vi "TimeInterpPose2d_CleanUp.vi"(11 "in TimeInterpPose":T1 {"Pose"."ROTATION"."SIN" format="%13.4f"; "Pose"."ROTATION"."COS" format="%13.4f"; "Pose"."ROTATION"."VALUE" format="%13.4f"; "Pose"."TRANSLATION"."Y" format="%14.3f"; "Pose"."TRANSLATION"."X" format="%14.3f"}) -> (0 "Error":bool, 3 "out TimeInterpPose":T1 {"Pose"."ROTATION"."SIN" format="%13.4f"; "Pose"."ROTATION"."COS" format="%13.4f"; "Pose"."ROTATION"."VALUE" format="%13.4f"; "Pose"."TRANSLATION"."Y" format="%14.3f"; "Pose"."TRANSLATION"."X" format="%14.3f"})   [LabVIEW 2019, in "Trajectory_Library.lvlib"]
doc: "Removes samples older than our current history size.\n\nInputs:\n - In TimeInterpPose2d -- Input data cluster.\n\nOutputs:\n - Out TimeInterpPose2d -- Updated data cluster.\n - Error -- Returns TRUE if an error occured."
uses:
  Trajectory_Library.lvlib
  TIME_INTERPOLATABLE_POSE2D.ctl
  POSE2D.ctl
  TRANSLATION2D.ctl
  ROTATION2D.ctl
  <vilib>/gmath/NI_Gmath.lvlib
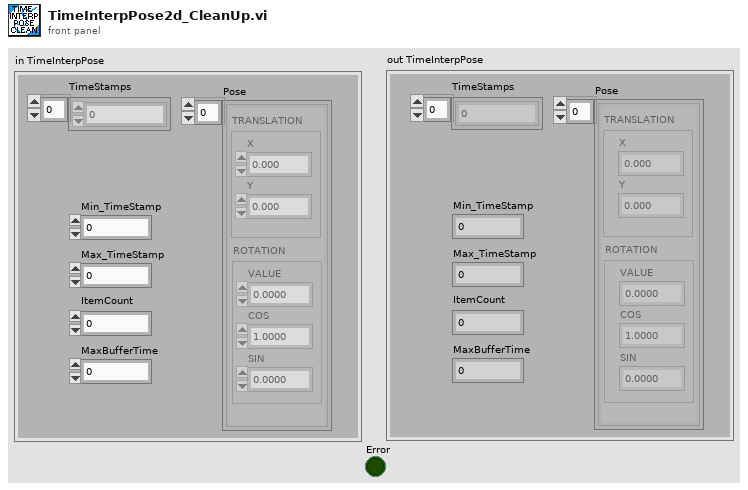
[diagram p1: front panel]
types:
  T1 = typedef "Trajectory_Library.lvlib/TIME_INTERPOLATABLE_POSE2D.ctl" = cluster{"TimeStamps":dbl[], "Pose":T2[], "Min_TimeStamp":dbl, "Max_TimeStamp":dbl, "ItemCount":i32, "MaxBufferTime":dbl}
  T2 = typedef "Trajectory_Library.lvlib/POSE2D.ctl" = cluster{"TRANSLATION":T3, "ROTATION":T4}
  T3 = typedef "Trajectory_Library.lvlib/TRANSLATION2D.ctl" = cluster{"X":dbl, "Y":dbl}
  T4 = typedef "Trajectory_Library.lvlib/ROTATION2D.ctl" = cluster{"VALUE":dbl, "COS":dbl, "SIN":dbl}
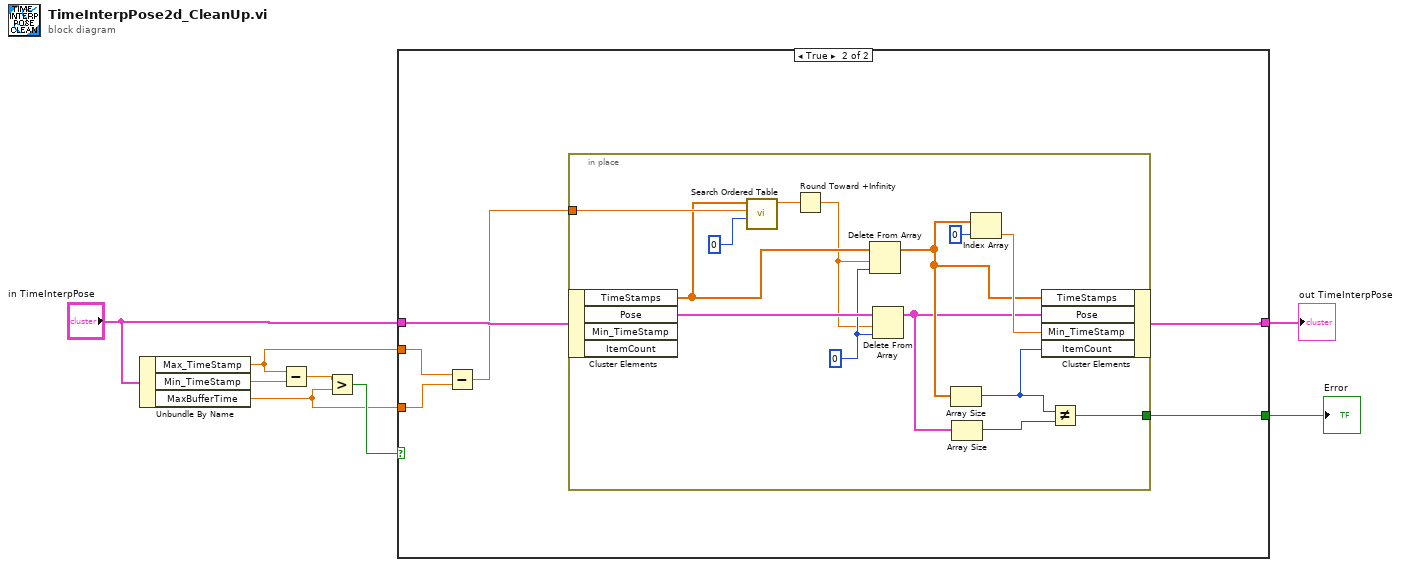
[diagram p0: block diagram]
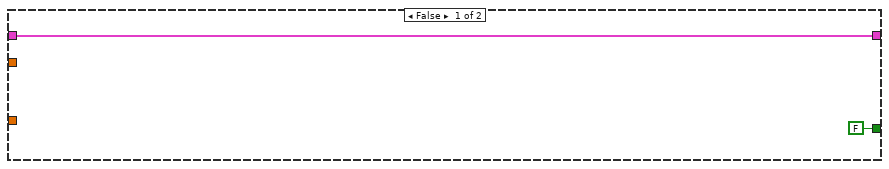
[diagram p2: hidden frame]
diagram:
  n1 = Unbundle By Name("in TimeInterpPose") -> ("Max_TimeStamp"=w3:dbl, "Min_TimeStamp"=w6:dbl, "MaxBufferTime"=w2:dbl)
  n2 = Subtract(x=w3, y=w6) -> (x-y=w5:dbl)
  n3 = Greater?(x=w5, y=w2) -> (0:w4:bool)
  n4 = case shown="True" w4 {
    tunnel: "in TimeInterpPose" -> [w10 w14]
    tunnel: [w10 w12] -> w8
    tunnel: w3 -> [_ w16]
    tunnel: w2 -> [_ w15]
    tunnel: [FALSE w11] -> w1
    frame False {
    }
    frame True {
      n5 = Subtract(x=w16, y=w15) -> (x-y=w13:dbl)
      n6 = in-place {
        in-place-border: w13 -> [w29]
        in-place-border: [w17] -> w11
        w25 = 0 ("index")
        n7 = in-place-cluster #1(w14) -> ("TimeStamps"=w28:dbl[], "Pose"=w27:T2[])  [unwired: 2 out]
        n8 = call <vilib>:"Search Ordered Table.vi"("starting index"=0, "x value"=w29, "ordered x array"=w28) -> ("fractional index"=w26:dbl)  [unwired: 8 in]
        n9 = Round Toward +Infinity(x=w26) -> (ceil(x): smallest int >= x=w24:dbl)
        n10 = Delete From Array(array=w28, length=w24, index=w25) -> (array with subset deleted=w21:dbl[])  [unwired: 1 out]
        n11 = Delete From Array(array=w27, length=w24, index=w25) -> (array with subset deleted=w20:T2[])  [unwired: 1 out]
        n12 = Array Size(array=w21) -> (size(s)=w19:i32)
        n13 = Array Size(array=w20) -> (size(s)=w18:i32)
        n14 = Index Array(array=w21, index=0) -> (element=w22:dbl)
        n15 = in-place-cluster #1("TimeStamps"=w21, "Pose"=w20, "Min_TimeStamp"=w22, "ItemCount"=w19) -> (w12:T1)
        n16 = Not Equal?(x=w19, y=w18) -> (x != y?=w17:bool)
      }
    }
  }
  "out TimeInterpPose" <- w8
  "Error" <- w1
